vi "write_param.vi"   [LabVIEW 2014]
uses:
  FT_HMI.llb/GLOBAL_PUMPS_PARAMS.vi
  FT_HMI.llb/GLOBAL_GEN.vi
  ADS.llb/Global DIOs.vi
types:
  T1 = cluster{"GENERAL":cluster{"NO ARTICLE":string, "DESIGNATION":string, "TENSION [V]":sgl, "FREQUENCE [Hz]":sgl, "BYPASS":bool}, "ST1_HT":cluster{"STATUS HT":bool, "TENSION ISOLATION [V]":sgl, "COURANT ISOLATION [mA]":sgl, "TEMPS DE MESURE [ms]":i32, "NO PROGRAMME":i32}, "ST2_ASPIRATION":cluster{"STATUS H ASP":bool, "TEMPS POMPAGE [ms]":i32, "STATUS CONTRE-PRESSION":bool, "HAUTEUR ASPIRATION [m]":sgl, "TEMPS DE MESURE ASP [ms]":i32, "STATUS PERTE ASP":bool, "PERTE ASPIRATION [mbar]":sgl, "TEMPS DE MESURE PERTE [ms] ":i32}, "ST3_ETANCHEITE":cluster{"STATUS":bool, "ETANCHEITE [mbar]":sgl, "TEMPS MISE SOUS PRESSION [ms]":i32, "TEMPS STABILISATION [ms]":i32, "TEMPS DE MESURE [ms]":i32}, "ST4-5_DEBIT":cluster{"STATUS QMAX":bool, "GRAND DEBIT":bool, "PUMPING_TIME  [ms]":i32, "DEBIT MIN [l/h]":sgl, "DEBIT MAX  [l/h]":sgl, "TEMPS DE MESURE QMAX [ms]":i32, "STATUS QTRAVAIL 1":bool, "DEBIT TRAVAIL 1 MIN [l/h]":sgl, "DEBIT TRAVAIL 1 MAX [l/h]":sgl, "PRESSION DE CONSIGNE 1 [bar]":sgl, "TEMPS DE REGLAGE PRESSION [ms]":i32, "TEMPS DE MESURE QTRAVAIL 1 [ms]":i32, "STATUS QTRAVAIL 2":bool, "DEBIT TRAVAIL 2 MIN [l/h]":sgl, "DEBIT TRAVAIL 2 MAX [l/h]":sgl, "PRESSION DE CONSIGNE 2 [bar]":sgl, "TEMPS DE MESURE QTRAVAIL 2 [ms]":i32, "STATUS CONSO":bool, "CONSOMMATION [A]":sgl, "TEMPS DE MESURE COURANT [ms]":i32}, "ST6_PRESSION":cluster{"STATUS PMAX":bool, "PUMPING TIME [ms]":i32, "PRESSION MIN [bar]":sgl, "TEMPS DE MESURE PMAX [ms]":i32, "STATUS PERTE PRESSION":bool, "PERTE PRESSION [mbar]":sgl, "TEMPS DE MESURE PERTE [ms]":i32}, "ST7_VIDANGE":cluster{"STATUS VIDANGE":bool, "TEMPS DE VIDANGE [ms] ":i32}, "ST8_IMPRESSION":cluster{"STATUS":bool, "ETIQUETTE":string}, "ST9_DECHARGEMENT":cluster{"STATUS":bool, "BOBINE A FIL":bool}, "DIVERS":cluster{"INDICE MODIF":string, "DATE MODIF":timestamp, "HISTORIQUE MODIF":string, "EMBOUT PRESSION":string, "EMBOUT ASPIRATION":string}}
  T2 = cluster{"ADS_GEN_GRAND_DEBIT_Header":i32, "ADS_GEN_BYPASS_Header":i32, "ADS_ST1_HT_NO_PROG_Header":i32, "ADS_ST2_TEMPS_POMPAGE_Header":i32, "ADS_ST2_CONTRE_PRESSION_Header":i32, "ADS_ST2_TEMPS_MESURE_Header":i32, "ADS_ST2_TEMPS_MESURE_PERTE_PRESSION_Header":i32, "ADS_ST3_TEMPS_MISE_SOUS_PRESSION_Header":i32, "ADS_ST3_TEMPS_STABILISATION_Header":i32, "ADS_ST3_TEMPS_MESURE_Header":i32, "ADS_ST45_TEMPS_POMPAGE_Header":i32, "ADS_ST45_TEMPS_MESURE_DEBIT_MAX_Header":i32, "ADS_ST45_TEMPS_REGLAGE_PRESSION_Header":i32, "ADS_ST45_TEMPS_MESURE_DEBIT_Header":i32, "ADS_ST45_PRESSION_CONSIGNE_Header":i32, "ADS_ST6_TEMPS_POMPAGE_Header":i32, "ADS_ST6_TEMPS_MESURE_Header":i32, "ADS_ST6_TEMPS_MESURE_PERTE_PRESSION_Header":i32, "ADS_ST7_TEMPS_SECHAGE_Header":i32, "ADS_ST9_BOBINE_A_FIL_Header":i32, "ADS_SAFETY_EM_State_Header":i32, "ADS_RESET_EMERGENCY_Header":i32, "ADS_FLAGS_SAFETY_Header":i32, "ADS_FLAGS_INIT_Header":i32, "ADS_FLAGS_AUTO_Header":i32, "ADS_PROG_STEPS_Header":i32, "ADS_GEMMA_Header":i32, "ADS_ST1_HT_OK_Header":i32, "ADS_ST2_VACUUM_Header":i32, "ADS_ST3_PRESSION_Header":i32, "ADS_ST3_DELTA_P_Header":i32, "ADS_ST45_QMAX_Header":i32, "ADS_ST45_Q_Header":i32, "ADS_ST45_PRESSURE_Header":i32, "ADS_ST45_VACUUM_Header":i32, "ADS_ST45_POIDS_Header":i32, "ADS_ST45_COURANT_Header":i32, "ADS_ST5_MODE_VIDANGE_Header":i16, "ADS_ST6_PRESSURE_Header":i16, "ADS_ST8_PRET_A_IMPRIMER_Header":i32, "ADS_ST8_IMPRESSION_OK_Header":i32, "ADS_ST9_DECHARGE_Header":i32, "ADS_SAFETY_RUN_Header":i32, "ADS_ST1_JIG_DISABLED_Header":i32, "ADS_ST2_JIG_DISABLED_Header":i32, "ADS_ST3_JIG_DISABLED_Header":i32, "ADS_ST4_5_JIG_DISABLED_Header":i32, "ADS_ST6_JIG_DISABLED_Header":i32, "ADS_ST7_JIG_DISABLED_Header":i32, "ADS_ST8_JIG_DISABLED_Header":i32, "ADS_ST9_JIG_DISABLED_Header":i32, "ADS_ST10_OPERATEUR1_START_Header":i32, "ADS_ST10_OPERATEUR2_START_Header":i32}
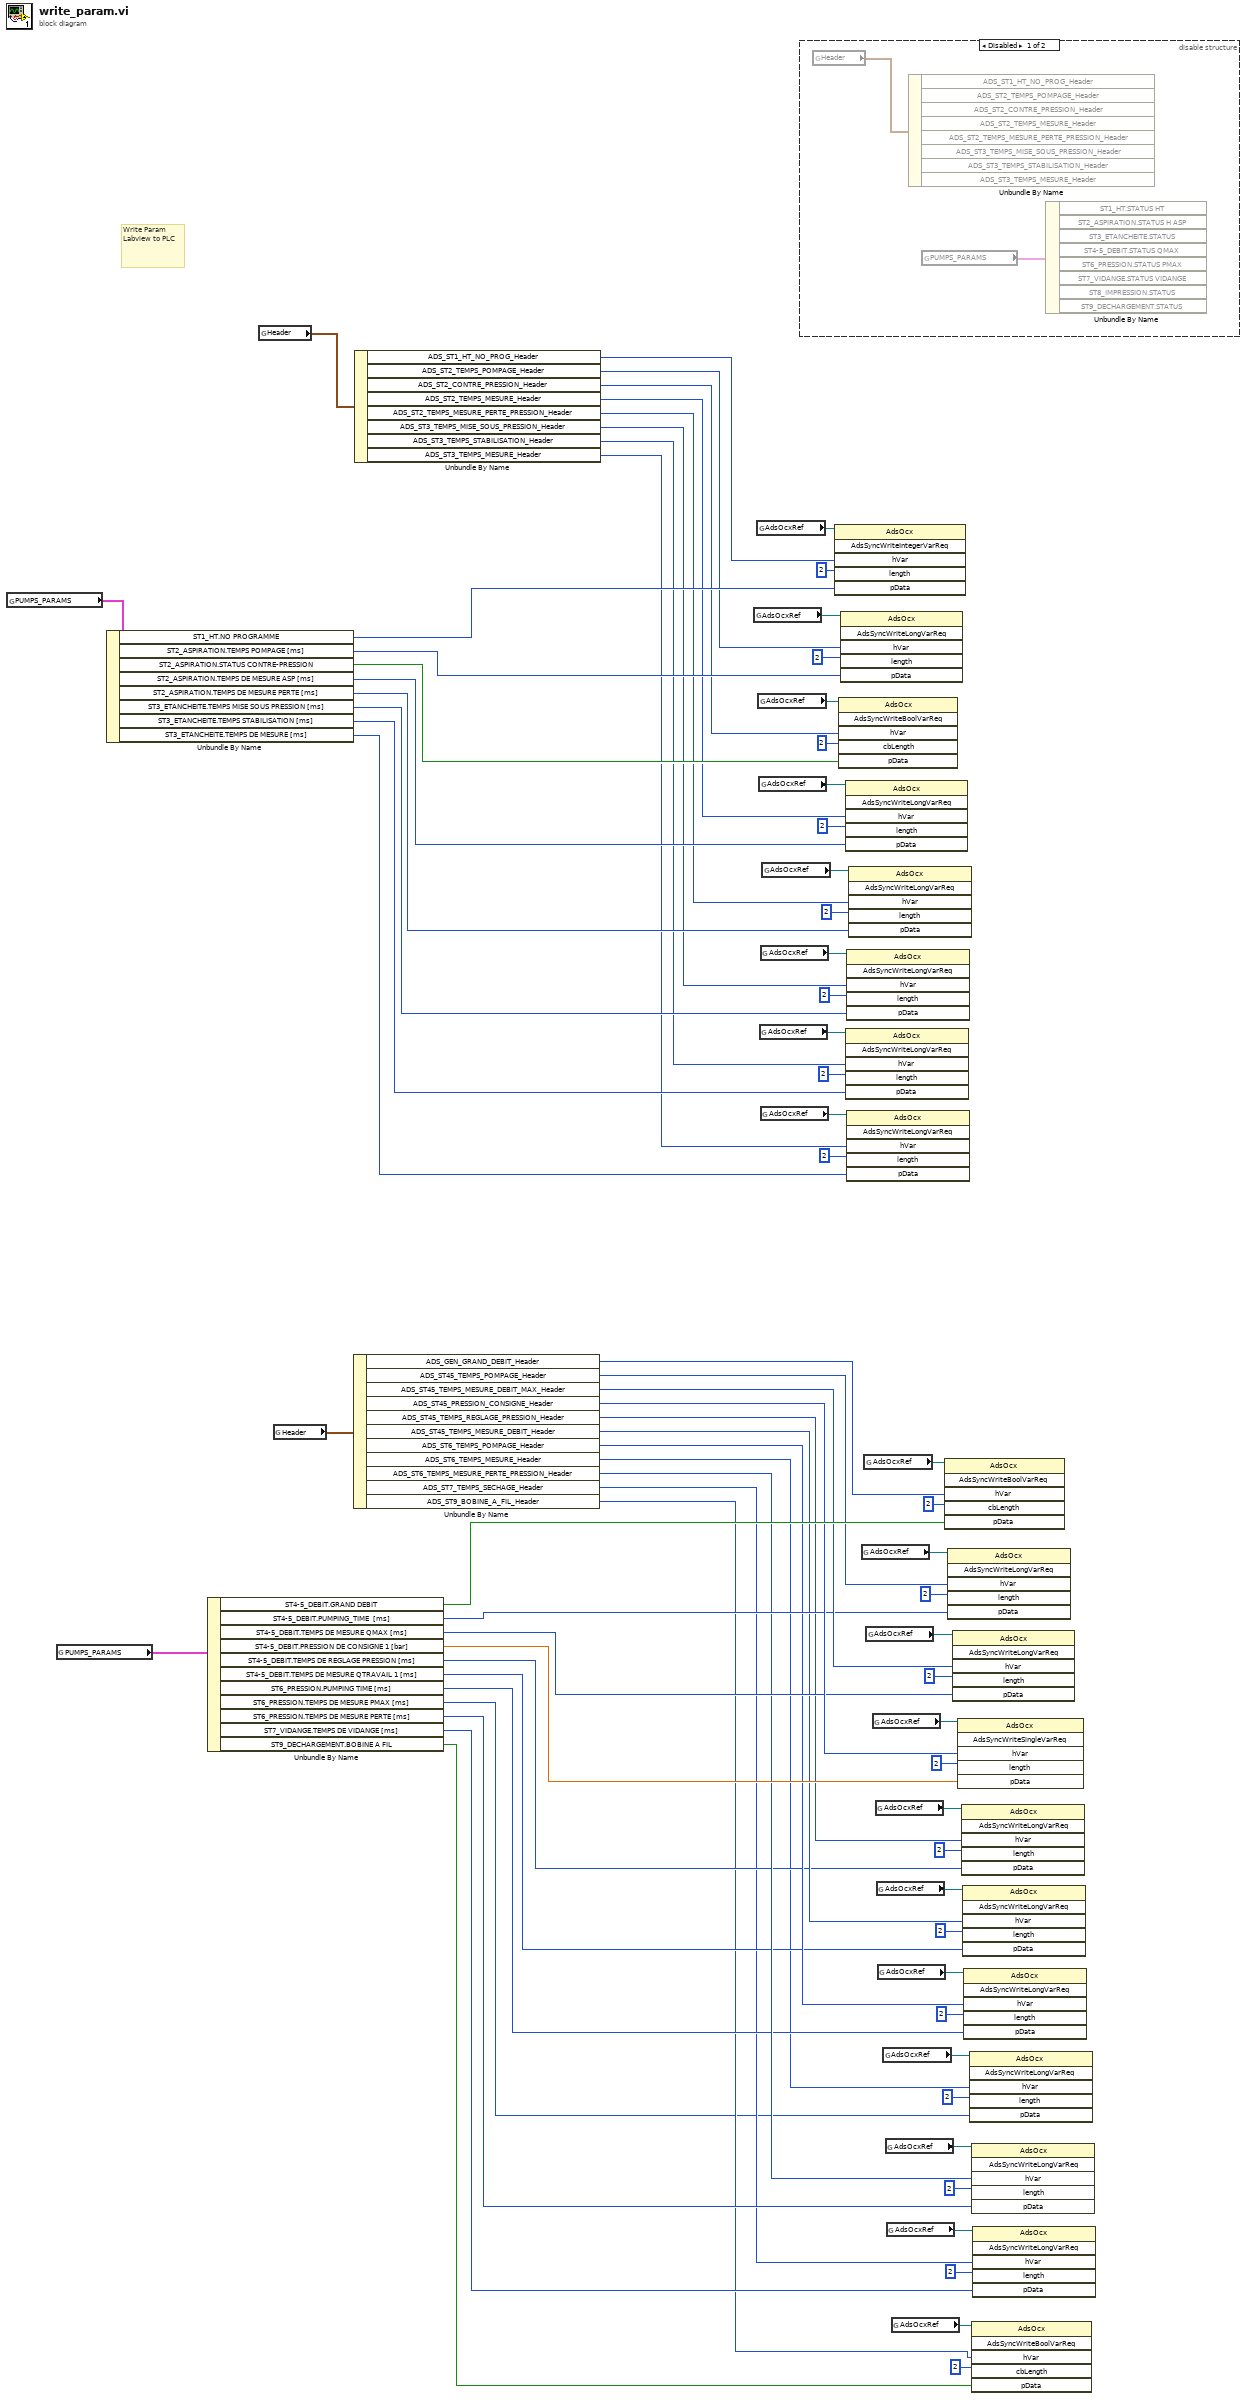
[diagram p0: block diagram]
diagram:
  # "Write Param Labview to PLC"
  n1 = global read "GLOBAL_PUMPS_PARAMS.vi" "PUMPS_PARAMS"() -> (w80:T1)
  n2 = global read "GLOBAL_PUMPS_PARAMS.vi" "PUMPS_PARAMS"() -> (w48:T1)
  n3 = Unbundle By Name(w80) -> ("ST1_HT.NO PROGRAMME"=w77:i32, "ST2_ASPIRATION.TEMPS POMPAGE [ms]"=w74:i32, "ST2_ASPIRATION.STATUS CONTRE-PRESSION"=w71:bool, "ST2_ASPIRATION.TEMPS DE MESURE ASP [ms]"=w66:i32, "ST2_ASPIRATION.TEMPS DE MESURE PERTE [ms]"=w65:i32, "ST3_ETANCHEITE.TEMPS MISE SOUS PRESSION [ms]"=w56:i32, "ST3_ETANCHEITE.TEMPS STABILISATION [ms]"=w52:i32, "ST3_ETANCHEITE.TEMPS DE MESURE [ms]"=w46:i32)
  n4 = Unbundle By Name(w48) -> ("ST4-5_DEBIT.GRAND DEBIT"=w39:bool, "ST4-5_DEBIT.PUMPING_TIME  [ms]"=w24:i32, "ST4-5_DEBIT.TEMPS DE MESURE QMAX [ms]"=w23:i32, "ST4-5_DEBIT.PRESSION DE CONSIGNE 1 [bar]"=w22:sgl, "ST4-5_DEBIT.TEMPS DE REGLAGE PRESSION [ms]"=w14:i32, "ST4-5_DEBIT.TEMPS DE MESURE QTRAVAIL 1 [ms]"=w13:i32, "ST6_PRESSION.PUMPING TIME [ms]"=w12:i32, "ST6_PRESSION.TEMPS DE MESURE PMAX [ms]"=w1:i32, "ST6_PRESSION.TEMPS DE MESURE PERTE [ms]"=w10:i32, "ST7_VIDANGE.TEMPS DE VIDANGE [ms]"=w11:i32, "ST9_DECHARGEMENT.BOBINE A FIL"=w9:bool)
  n5 = global read "Global DIOs.vi" "Header"() -> (w64:T2)
  n6 = global read "Global DIOs.vi" "Header"() -> (w45:T2)
  n7 = Unbundle By Name(w45) -> ("ADS_GEN_GRAND_DEBIT_Header"=w40:i32, "ADS_ST45_TEMPS_POMPAGE_Header"=w38:i32, "ADS_ST45_TEMPS_MESURE_DEBIT_MAX_Header"=w26:i32, "ADS_ST45_PRESSION_CONSIGNE_Header"=w25:i32, "ADS_ST45_TEMPS_REGLAGE_PRESSION_Header"=w21:i32, "ADS_ST45_TEMPS_MESURE_DEBIT_Header"=w20:i32, "ADS_ST6_TEMPS_POMPAGE_Header"=w19:i32, "ADS_ST6_TEMPS_MESURE_Header"=w2:i32, "ADS_ST6_TEMPS_MESURE_PERTE_PRESSION_Header"=w15:i32, "ADS_ST7_TEMPS_SECHAGE_Header"=w7:i32, "ADS_ST9_BOBINE_A_FIL_Header"=w8:i32)
  n8 = Unbundle By Name(w64) -> ("ADS_ST1_HT_NO_PROG_Header"=w63:i32, "ADS_ST2_TEMPS_POMPAGE_Header"=w62:i32, "ADS_ST2_CONTRE_PRESSION_Header"=w61:i32, "ADS_ST2_TEMPS_MESURE_Header"=w60:i32, "ADS_ST2_TEMPS_MESURE_PERTE_PRESSION_Header"=w59:i32, "ADS_ST3_TEMPS_MISE_SOUS_PRESSION_Header"=w55:i32, "ADS_ST3_TEMPS_STABILISATION_Header"=w51:i32, "ADS_ST3_TEMPS_MESURE_Header"=w47:i32)
  n9 = global read "GLOBAL_GEN.vi" "AdsOcxRef"() -> (w75:refnum<k7>)
  n10 = global read "GLOBAL_GEN.vi" "AdsOcxRef"() -> (w78:refnum<k7>)
  n11 = global read "GLOBAL_GEN.vi" "AdsOcxRef"() -> (w72:refnum<k7>)
  n12 = global read "GLOBAL_GEN.vi" "AdsOcxRef"() -> (w69:refnum<k7>)
  n13 = global read "GLOBAL_GEN.vi" "AdsOcxRef"() -> (w53:refnum<k7>)
  n14 = global read "GLOBAL_GEN.vi" "AdsOcxRef"() -> (w57:refnum<k7>)
  n15 = global read "GLOBAL_GEN.vi" "AdsOcxRef"() -> (w49:refnum<k7>)
  n16 = global read "GLOBAL_GEN.vi" "AdsOcxRef"() -> (w67:refnum<k7>)
  n17 = disable-structure shown="Disabled" {
    frame Disabled {
      n18 = global read "Global DIOs.vi" "Header"() -> (w81:T2)
      n19 = Unbundle By Name(w81) -> ()  [unwired: 8 out]
      n20 = global read "GLOBAL_PUMPS_PARAMS.vi" "PUMPS_PARAMS"() -> (w82:T1)
      n21 = Unbundle By Name(w82) -> ()  [unwired: 8 out]
    }
    frame Enabled {
    }
  }
  n22 = invoke class="AdsOcx" method="AdsSyncWriteIntegerVarReq"(reference=w78, "hVar"=w63, "length"=2 ("phConnect"), "pData"=w77) -> ()  [unwired: 2 in, 6 out]
  n23 = invoke class="AdsOcx" method="AdsSyncWriteBoolVarReq"(reference=w72, "hVar"=w61, "cbLength"=2 ("phConnect"), "pData"=w71) -> ()  [unwired: 2 in, 6 out]
  n24 = invoke class="AdsOcx" method="AdsSyncWriteLongVarReq"(reference=w75, "hVar"=w62, "length"=2 ("phConnect"), "pData"=w74) -> ()  [unwired: 2 in, 6 out]
  n25 = invoke class="AdsOcx" method="AdsSyncWriteLongVarReq"(reference=w69, "hVar"=w60, "length"=2 ("phConnect"), "pData"=w66) -> ()  [unwired: 2 in, 6 out]
  n26 = invoke class="AdsOcx" method="AdsSyncWriteLongVarReq"(reference=w53, "hVar"=w51, "length"=2 ("phConnect"), "pData"=w52) -> ()  [unwired: 2 in, 6 out]
  n27 = invoke class="AdsOcx" method="AdsSyncWriteLongVarReq"(reference=w57, "hVar"=w55, "length"=2 ("phConnect"), "pData"=w56) -> ()  [unwired: 2 in, 6 out]
  n28 = invoke class="AdsOcx" method="AdsSyncWriteLongVarReq"(reference=w49, "hVar"=w47, "length"=2 ("phConnect"), "pData"=w46) -> ()  [unwired: 2 in, 6 out]
  n29 = invoke class="AdsOcx" method="AdsSyncWriteLongVarReq"(reference=w67, "hVar"=w59, "length"=2 ("phConnect"), "pData"=w65) -> ()  [unwired: 2 in, 6 out]
  n30 = global read "GLOBAL_GEN.vi" "AdsOcxRef"() -> (w43:refnum<k7>)
  n31 = global read "GLOBAL_GEN.vi" "AdsOcxRef"() -> (w41:refnum<k7>)
  n32 = global read "GLOBAL_GEN.vi" "AdsOcxRef"() -> (w36:refnum<k7>)
  n33 = global read "GLOBAL_GEN.vi" "AdsOcxRef"() -> (w34:refnum<k7>)
  n34 = global read "GLOBAL_GEN.vi" "AdsOcxRef"() -> (w32:refnum<k7>)
  n35 = global read "GLOBAL_GEN.vi" "AdsOcxRef"() -> (w30:refnum<k7>)
  n36 = global read "GLOBAL_GEN.vi" "AdsOcxRef"() -> (w29:refnum<k7>)
  n37 = global read "GLOBAL_GEN.vi" "AdsOcxRef"() -> (w27:refnum<k7>)
  n38 = global read "GLOBAL_GEN.vi" "AdsOcxRef"() -> (w16:refnum<k7>)
  n39 = global read "GLOBAL_GEN.vi" "AdsOcxRef"() -> (w6:refnum<k7>)
  n40 = global read "GLOBAL_GEN.vi" "AdsOcxRef"() -> (w3:refnum<k7>)
  n41 = invoke class="AdsOcx" method="AdsSyncWriteBoolVarReq"(reference=w41, "hVar"=w40, "cbLength"=2 ("phConnect"), "pData"=w39) -> ()  [unwired: 2 in, 6 out]
  n42 = invoke class="AdsOcx" method="AdsSyncWriteLongVarReq"(reference=w43, "hVar"=w38, "length"=2 ("phConnect"), "pData"=w24) -> ()  [unwired: 2 in, 6 out]
  n43 = invoke class="AdsOcx" method="AdsSyncWriteLongVarReq"(reference=w36, "hVar"=w26, "length"=2 ("phConnect"), "pData"=w23) -> ()  [unwired: 2 in, 6 out]
  n44 = invoke class="AdsOcx" method="AdsSyncWriteSingleVarReq"(reference=w34, "hVar"=w25, "length"=2 ("phConnect"), "pData"=w22) -> ()  [unwired: 2 in, 6 out]
  n45 = invoke class="AdsOcx" method="AdsSyncWriteLongVarReq"(reference=w32, "hVar"=w21, "length"=2 ("phConnect"), "pData"=w14) -> ()  [unwired: 2 in, 6 out]
  n46 = invoke class="AdsOcx" method="AdsSyncWriteLongVarReq"(reference=w30, "hVar"=w20, "length"=2 ("phConnect"), "pData"=w13) -> ()  [unwired: 2 in, 6 out]
  n47 = invoke class="AdsOcx" method="AdsSyncWriteLongVarReq"(reference=w29, "hVar"=w19, "length"=2 ("phConnect"), "pData"=w12) -> ()  [unwired: 2 in, 6 out]
  n48 = invoke class="AdsOcx" method="AdsSyncWriteLongVarReq"(reference=w27, "hVar"=w2, "length"=2 ("phConnect"), "pData"=w1) -> ()  [unwired: 2 in, 6 out]
  n49 = invoke class="AdsOcx" method="AdsSyncWriteLongVarReq"(reference=w16, "hVar"=w15, "length"=2 ("phConnect"), "pData"=w10) -> ()  [unwired: 2 in, 6 out]
  n50 = invoke class="AdsOcx" method="AdsSyncWriteBoolVarReq"(reference=w3, "hVar"=w8, "cbLength"=2 ("phConnect"), "pData"=w9) -> ()  [unwired: 2 in, 6 out]
  n51 = invoke class="AdsOcx" method="AdsSyncWriteLongVarReq"(reference=w6, "hVar"=w7, "length"=2 ("phConnect"), "pData"=w11) -> ()  [unwired: 2 in, 6 out]
